vi "DriverStationGetData.vi"   [LabVIEW 2019]
uses:
  <vilib>/Rock Robotics/Network Tables/NT Read Boolean.vi
  dsdata.vi
  <vilib>/Rock Robotics/Network Tables/NT Read Number.vi
  sensors.vi
  <vilib>/Rock Robotics/Network Tables/NT Read String.vi
  refnums.vi
  <vilib>/Rock Robotics/WPI/Utilities/WPI_GetSetVariantRefNum.vi
types:
  T1 = typedef "WPI_JoystickDevRef.ctl" = cluster{"Device":T2}
  T2 = typedef "WPI_JoystickDeviceEnum.ctl" = enum16{"USB 0", "USB 1", "USB 2", "USB 3", "USB 4", "USB 5"}
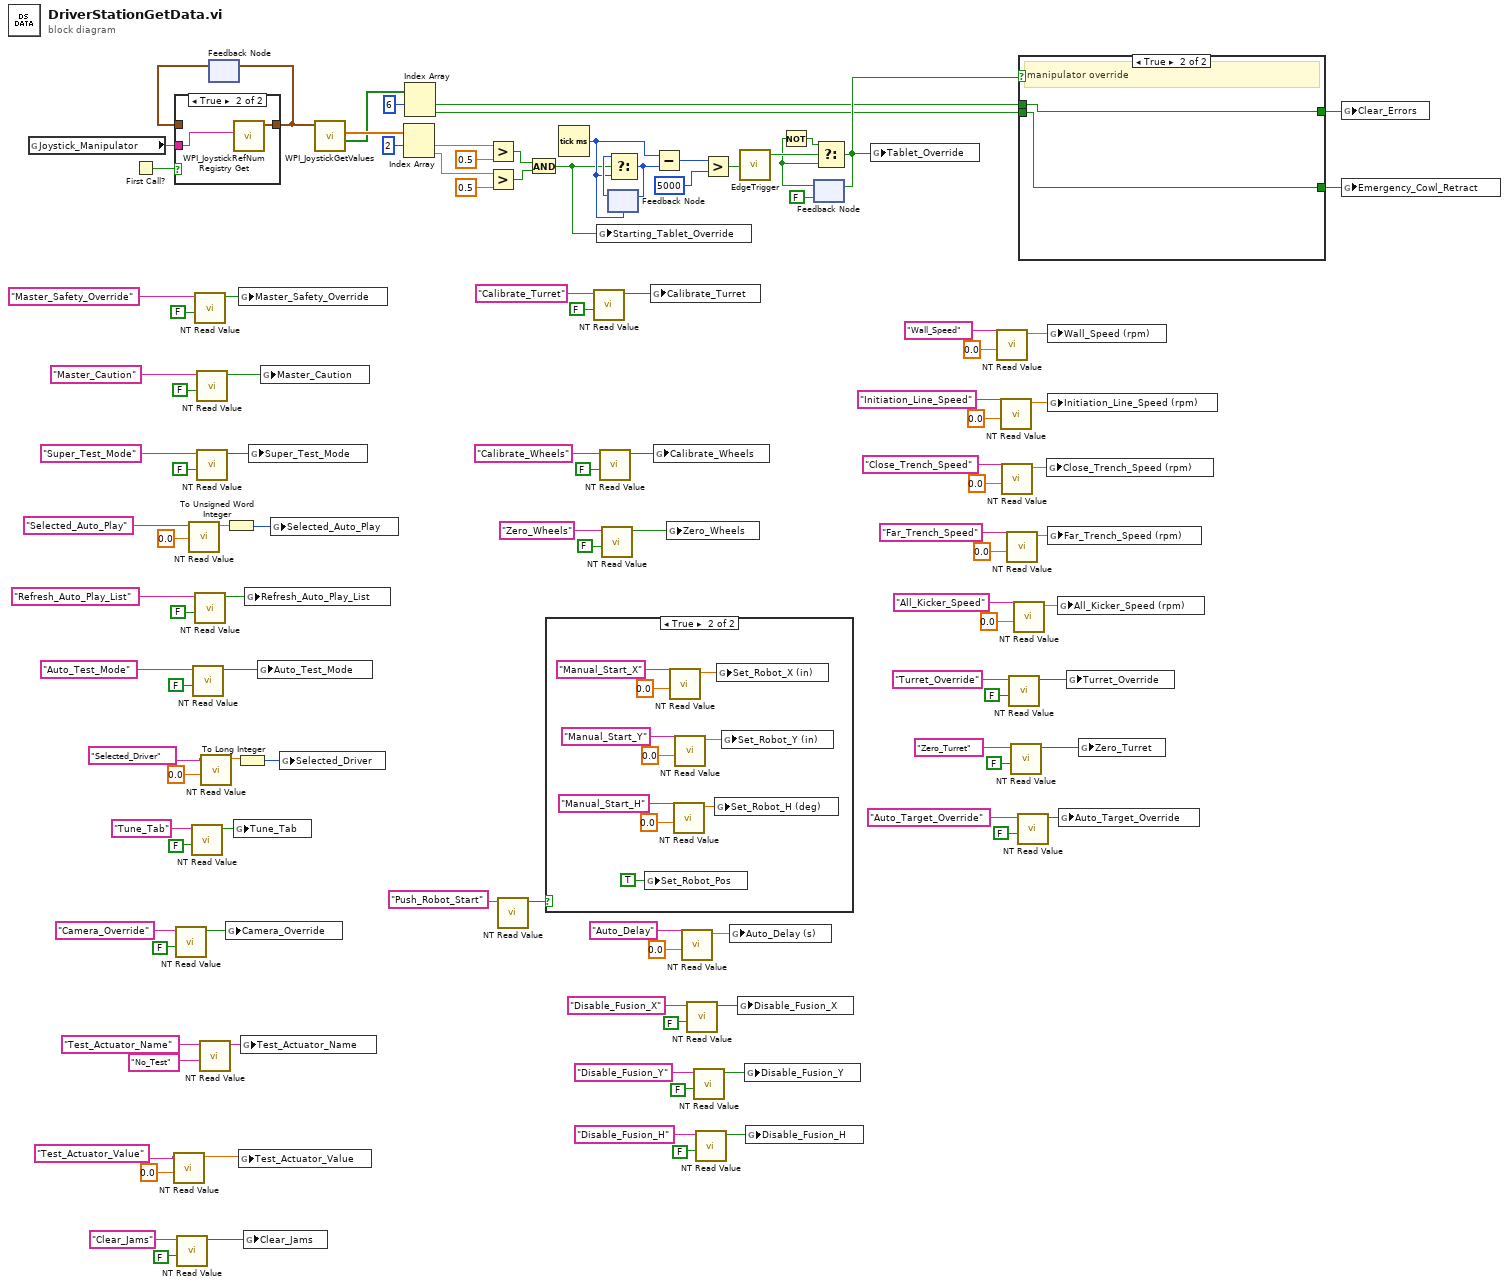
[diagram p0: block diagram]
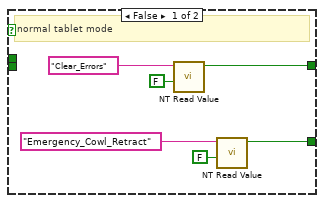
[diagram p2: hidden frame]
diagram:
  n1 = global read "refnums.vi" "Joystick_Manipulator"() -> (w33:string)
  n2 = First Call?() -> (First Call?: T/F=w36:bool)
  n3 = call-poly <vilib>:"NT Read Value.vi"("Default Value"=0.0, "Name"="Test_Actuator_Value" ("refnum name")) -> ("Numeric"=w43:dbl)  [unwired: 8 in, 1 out]
  n4 = call-poly <vilib>:"NT Read Value.vi"("Default Value"=FALSE, "Name"="Camera_Override" ("refnum name")) -> ("Boolean"=w79:bool)  [unwired: 8 in, 1 out]
  n5 = call-poly <vilib>:"NT Read Value.vi"("Default Value"=FALSE, "Name"="Clear_Jams" ("refnum name")) -> ("Boolean"=w1:bool)  [unwired: 8 in, 1 out]
  n6 = call-poly <vilib>:"NT Read Value.vi"("Default Value"=0.0, "Name"="Selected_Auto_Play" ("refnum name")) -> ("Numeric"=w107:dbl)  [unwired: 8 in, 1 out]
  n7 = call-poly <vilib>:"NT Read Value.vi"("Default Value"=FALSE, "Name"="Tune_Tab" ("refnum name")) -> ("Boolean"=w100:bool)  [unwired: 8 in, 1 out]
  n8 = call-poly <vilib>:"NT Read Value.vi"("Default Value"=FALSE, "Name"="Auto_Test_Mode" ("refnum name")) -> ("Boolean"=w82:bool)  [unwired: 8 in, 1 out]
  n9 = call-poly <vilib>:"NT Read Value.vi"("Default Value"=FALSE, "Name"="Master_Safety_Override" ("refnum name")) -> ("Boolean"=w85:bool)  [unwired: 8 in, 1 out]
  n10 = call-poly <vilib>:"NT Read Value.vi"("Default Value"=FALSE, "Name"="Refresh_Auto_Play_List" ("refnum name")) -> ("Boolean"=w110:bool)  [unwired: 8 in, 1 out]
  n11 = call-poly <vilib>:"NT Read Value.vi"("Default Value"=FALSE, "Name"="Master_Caution" ("refnum name")) -> ("Boolean"=w4:bool)  [unwired: 8 in, 1 out]
  n12 = call-poly <vilib>:"NT Read Value.vi"("Default Value"=FALSE, "Name"="Super_Test_Mode" ("refnum name")) -> ("Boolean"=w113:bool)  [unwired: 8 in, 1 out]
  n13 = call-poly <vilib>:"NT Read Value.vi"("Default Value"="No_Test", "Name"="Test_Actuator_Name" ("refnum name")) -> ("String"=w47:string)  [unwired: 8 in, 1 out]
  n14 = call-poly <vilib>:"NT Read Value.vi"("Default Value"=0.0, "Name"="Selected_Driver" ("refnum name")) -> ("Numeric"=w102:dbl)  [unwired: 8 in, 1 out]
  n15 = feedback #1() -> (w35:T1)  [unwired: 1 in]
  n16 = case shown="True" w36 {
    tunnel: [w116 w118] -> w34
    tunnel: w35 -> [w116 _]
    tunnel: w33 -> [_ w117]
    frame False {
    }
    frame True {
      n17 = call <vilib>:"WPI_JoystickRefNum Registry Get.vi"("refnum name"=w117) -> ("JoystickDevRef"=w118:T1)  [unwired: 9 in, 1 out]
    }
  }
  n18 = feedback-in #1(w34) -> ()
  n19 = To Unsigned Word Integer(number=w107) -> (unsigned 16bit integer=w106:u16)
  n20 = global write "dsdata.vi" "Camera_Override"(w79) -> ()
  n21 = global write "dsdata.vi" "Tune_Tab"(w100) -> ()
  n22 = To Long Integer(number=w102) -> (32bit integer=w99:i32)
  n23 = global write "dsdata.vi" "Master_Safety_Override"(w85) -> ()
  n24 = global write "dsdata.vi" "Test_Actuator_Value"(w43) -> ()
  n25 = global write "dsdata.vi" "Test_Actuator_Name"(w47) -> ()
  n26 = global write "dsdata.vi" "Clear_Jams"(w1) -> ()
  n27 = global write "dsdata.vi" "Refresh_Auto_Play_List"(w110) -> ()
  n28 = global write "dsdata.vi" "Super_Test_Mode"(w113) -> ()
  n29 = global write "dsdata.vi" "Auto_Test_Mode"(w82) -> ()
  n30 = global write "dsdata.vi" "Master_Caution"(w4) -> ()
  n31 = global write "dsdata.vi" "Selected_Auto_Play"(w106) -> ()
  n32 = global write "dsdata.vi" "Selected_Driver"(w99) -> ()
  n33 = call <vilib>:"WPI_JoystickGetValues.vi"("JoystickDevRef"=w34) -> ("Buttons"=w11:bool[], "Axes"=w32:dbl[])  [unwired: 6 in, 3 out]
  n34 = Index Array(array=w32, index #1=2 ("index")) -> (element #1=w18:dbl, element #2=w17:dbl)  [unwired: 1 in]
  n35 = Index Array(array=w11, index #1=6 ("index")) -> (element #1=w9:bool, element #2=w8:bool)  [unwired: 1 in]
  n36 = Greater?(x=w18, y=0.5) -> (0:w19:bool)
  n37 = Greater?(x=w17, y=0.5) -> (0:w15:bool)
  n38 = call-poly <vilib>:"NT Read Value.vi"("Name"="Push_Robot_Start" ("refnum name")) -> ("Boolean"=w91:bool)  [unwired: 9 in, 1 out]
  n39 = And(x=w19, y=w15) -> (x .and. y?=w7:bool)
  n40 = case shown="True" w91 {
    frame False {
    }
    frame True {
      n41 = global write "sensors.vi" "Set_Robot_Pos"(TRUE ("Set_Robot_Pos")) -> ()
      n42 = call-poly <vilib>:"NT Read Value.vi"("Default Value"=0.0, "Name"="Manual_Start_X" ("refnum name")) -> ("Numeric"=w126:dbl)  [unwired: 8 in, 1 out]
      n43 = call-poly <vilib>:"NT Read Value.vi"("Default Value"=0.0, "Name"="Manual_Start_H" ("refnum name")) -> ("Numeric"=w120:dbl)  [unwired: 8 in, 1 out]
      n44 = call-poly <vilib>:"NT Read Value.vi"("Default Value"=0.0, "Name"="Manual_Start_Y" ("refnum name")) -> ("Numeric"=w123:dbl)  [unwired: 8 in, 1 out]
      n45 = global write "sensors.vi" "Set_Robot_H (deg)"(w120) -> ()
      n46 = global write "sensors.vi" "Set_Robot_X (in)"(w126) -> ()
      n47 = global write "sensors.vi" "Set_Robot_Y (in)"(w123) -> ()
    }
  }
  n48 = Tick Count (ms)() -> (millisecond timer value=w27:u32)
  n49 = call-poly <vilib>:"NT Read Value.vi"("Default Value"=FALSE, "Name"="Calibrate_Turret" ("refnum name")) -> ("Boolean"=w52:bool)  [unwired: 8 in, 1 out]
  n50 = global write "dsdata.vi" "Starting_Tablet_Override"(w7) -> ()
  n51 = call-poly <vilib>:"NT Read Value.vi"("Default Value"=FALSE, "Name"="Calibrate_Wheels" ("refnum name")) -> ("Boolean"=w96:bool)  [unwired: 8 in, 1 out]
  n52 = call-poly <vilib>:"NT Read Value.vi"("Default Value"=FALSE, "Name"="Zero_Wheels" ("refnum name")) -> ("Boolean"=w93:bool)  [unwired: 8 in, 1 out]
  n53 = feedback #2(w27) -> (w29:u32)
  n54 = Select(t=w29, s=w7, f=w27) -> (s? t:f=w28:u32)
  n55 = feedback-in #2(w28) -> ()
  n56 = global write "dsdata.vi" "Calibrate_Turret"(w52) -> ()
  n57 = Subtract(x=w27, y=w28) -> (x-y=w26:u32)
  n58 = global write "dsdata.vi" "Calibrate_Wheels"(w96) -> ()
  n59 = global write "dsdata.vi" "Zero_Wheels"(w93) -> ()
  n60 = call-poly <vilib>:"NT Read Value.vi"("Default Value"=0.0, "Name"="Auto_Delay" ("refnum name")) -> ("Numeric"=w88:dbl)  [unwired: 8 in, 1 out]
  n61 = call-poly <vilib>:"NT Read Value.vi"("Default Value"=FALSE, "Name"="Disable_Fusion_X" ("refnum name")) -> ("Boolean"=w76:bool)  [unwired: 8 in, 1 out]
  n62 = call-poly <vilib>:"NT Read Value.vi"("Default Value"=FALSE, "Name"="Disable_Fusion_Y" ("refnum name")) -> ("Boolean"=w73:bool)  [unwired: 8 in, 1 out]
  n63 = call-poly <vilib>:"NT Read Value.vi"("Default Value"=FALSE, "Name"="Disable_Fusion_H" ("refnum name")) -> ("Boolean"=w70:bool)  [unwired: 8 in, 1 out]
  n64 = Greater?(x=w26, y=u32 5000) -> (0:w24:bool)
  n65 = global write "dsdata.vi" "Auto_Delay (s)"(w88) -> ()
  n66 = global write "dsdata.vi" "Disable_Fusion_X"(w76) -> ()
  n67 = call "EdgeTrigger.vi"("Input Signal"=w24) -> ("Rising Edge Trigger"=w23:bool)  [unwired: 2 out]
  n68 = global write "dsdata.vi" "Disable_Fusion_Y"(w73) -> ()
  n69 = global write "dsdata.vi" "Disable_Fusion_H"(w70) -> ()
  n70 = feedback #3(FALSE) -> (w20:bool)
  n71 = Not(x=w20) -> (.not. x?=w22:bool)
  n72 = Select(t=w22, s=w23, f=w20) -> (s? t:f=w13:bool)
  n73 = feedback-in #3(w13) -> ()
  n74 = global write "dsdata.vi" "Tablet_Override"(w13) -> ()
  n75 = call-poly <vilib>:"NT Read Value.vi"("Default Value"=0.0, "Name"="Wall_Speed" ("refnum name")) -> ("Numeric"=w64:dbl)  [unwired: 8 in, 1 out]
  n76 = call-poly <vilib>:"NT Read Value.vi"("Default Value"=0.0, "Name"="Initiation_Line_Speed" ("refnum name")) -> ("Numeric"=w67:dbl)  [unwired: 8 in, 1 out]
  n77 = call-poly <vilib>:"NT Read Value.vi"("Default Value"=0.0, "Name"="Close_Trench_Speed" ("refnum name")) -> ("Numeric"=w61:dbl)  [unwired: 8 in, 1 out]
  n78 = call-poly <vilib>:"NT Read Value.vi"("Default Value"=0.0, "Name"="Far_Trench_Speed" ("refnum name")) -> ("Numeric"=w58:dbl)  [unwired: 8 in, 1 out]
  n79 = call-poly <vilib>:"NT Read Value.vi"("Default Value"=FALSE, "Name"="Turret_Override" ("refnum name")) -> ("Boolean"=w49:bool)  [unwired: 8 in, 1 out]
  n80 = call-poly <vilib>:"NT Read Value.vi"("Default Value"=FALSE, "Name"="Zero_Turret" ("refnum name")) -> ("Boolean"=w40:bool)  [unwired: 8 in, 1 out]
  n81 = call-poly <vilib>:"NT Read Value.vi"("Default Value"=0.0, "Name"="All_Kicker_Speed" ("refnum name")) -> ("Numeric"=w55:dbl)  [unwired: 8 in, 1 out]
  n82 = call-poly <vilib>:"NT Read Value.vi"("Default Value"=FALSE, "Name"="Auto_Target_Override" ("refnum name")) -> ("Boolean"=w37:bool)  [unwired: 8 in, 1 out]
  n83 = case shown="True" w13 {
    tunnel: [w132 w136] -> w14
    tunnel: [w129 w135] -> w12
    tunnel: w9 -> [_ w136]
    tunnel: w8 -> [_ w135]
    frame False {
      # "normal tablet mode"
      n84 = call-poly <vilib>:"NT Read Value.vi"("Default Value"=FALSE, "Name"="Clear_Errors" ("refnum name")) -> ("Boolean"=w132:bool)  [unwired: 8 in, 1 out]
      n85 = call-poly <vilib>:"NT Read Value.vi"("Default Value"=FALSE, "Name"="Emergency_Cowl_Retract" ("refnum name")) -> ("Boolean"=w129:bool)  [unwired: 8 in, 1 out]
    }
    frame True {
      # "manipulator override"
    }
  }
  n86 = global write "dsdata.vi" "Close_Trench_Speed (rpm)"(w61) -> ()
  n87 = global write "dsdata.vi" "Wall_Speed (rpm)"(w64) -> ()
  n88 = global write "dsdata.vi" "Initiation_Line_Speed (rpm)"(w67) -> ()
  n89 = global write "dsdata.vi" "Far_Trench_Speed (rpm)"(w58) -> ()
  n90 = global write "dsdata.vi" "All_Kicker_Speed (rpm)"(w55) -> ()
  n91 = global write "dsdata.vi" "Auto_Target_Override"(w37) -> ()
  n92 = global write "dsdata.vi" "Turret_Override"(w49) -> ()
  n93 = global write "dsdata.vi" "Zero_Turret"(w40) -> ()
  n94 = global write "dsdata.vi" "Clear_Errors"(w14) -> ()
  n95 = global write "dsdata.vi" "Emergency_Cowl_Retract"(w12) -> ()
